vi "Class Name.vi"(8 "error in (no error)":errorcluster, 11 "Send in":refnum<class "Send.lvclass">) -> (0 "error out":errorcluster, 2 "Class Name":string, 3 "Send out":refnum<class "Send.lvclass">)   [LabVIEW 2011, in "Messenging.lvlib" / "Send.lvclass"]
uses:
  Send.lvclass
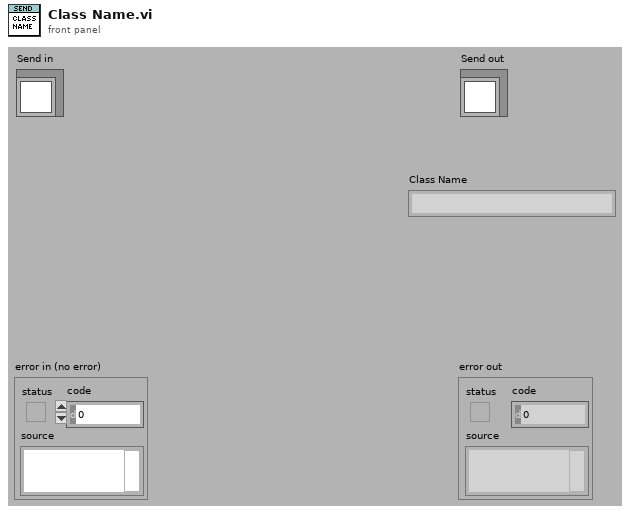
[diagram p1: front panel]
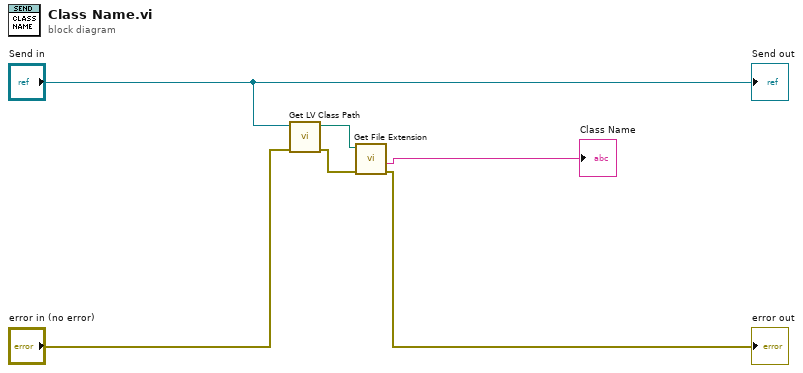
[diagram p0: block diagram]
diagram:
  n1 = call <vilib>:"Get LV Class Path.vi"("error in (no error)"="error in (no error)", "object"="Send in") -> ("error out"=w4:errorcluster, "class path"=w5:path)  [unwired: 8 out]
  n2 = call <vilib>:"Get File Extension.vi"("error in (no error)"=w4, "file"=w5) -> ("error out"=→"error out":errorcluster, "filename without extension"=→"Class Name":string)  [unwired: 8 out]
  "Send out" <- "Send in"
